vi "parseEnumerationString.vi"(8 "error in (no error)":errorcluster, 10 "IDLConstants":string, 11 "Enumeration in":refnum<class "Enumeration.lvclass">) -> (0 "error out":errorcluster, 3 "Enumeration out":refnum<class "Enumeration.lvclass">)   [LabVIEW 2016, in "Enumeration.lvclass"]
uses:
  Enumeration.lvclass
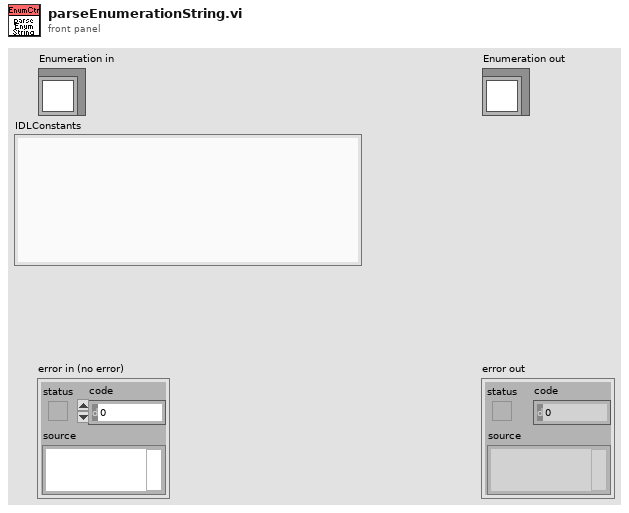
[diagram p1: front panel]
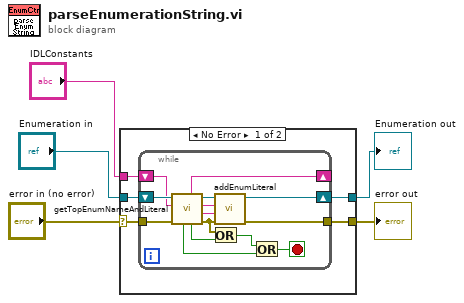
[diagram p0: block diagram]
diagram:
  n1 = case shown="No Error" "error in (no error)" {
    selector: "error in (no error)" -> [w10 w26]
    tunnel: [w9 w26] -> w4
    tunnel: [w7 w25] -> w2
    tunnel: "Enumeration in" -> [w8 w25]
    tunnel: "IDLConstants" -> [w6 _]
    frame No Error {
      n2 = while {
        shift-right: [w22] -> _
        shift-left: w6 -> [w23]
        tunnel: w10 -> [w21]
        tunnel: [w18] -> w9
        shift-right: [w17] -> w7
        shift-left: w8 -> [w24]
        stop <- w11 stop-if-true
        n3 = call "getTopEnumNameAndLiteral.vi"("error in (no error)"=w21, "IDLConstants"=w23, "Enumeration in"=w24) -> ("error out"=w19:errorcluster, "enumerationLiteral"=w14:string, "enumName"=w15:string, "Enumeration out"=w16:refnum<class "Enumeration.lvclass">, "endOfString"=w20:bool, "restOfString"=w22:string, "noMatch"=w12:bool)  [unwired: 2 in]
        n4 = Or(x=w19, y=w20) -> (x .or. y?=w13:bool)
        n5 = call "addEnumLiteral.vi"("error in (no error)"=w19, "enumerationLiteral"=w14, "enumName"=w15, "Enumeration in"=w16) -> ("error out"=w18:errorcluster, "Enumeration out"=w17:refnum<class "Enumeration.lvclass">)  [unwired: 6 in]
        n6 = Or(x=w13, y=w12) -> (x .or. y?=w11:bool)
      }
    }
    frame Error {
    }
  }
  "error out" <- w4
  "Enumeration out" <- w2
